vi "Configure Trigger Source.vi"(5 "Trigger Holdoff (0)":dbl min=0.0 max=1.0, 6 "Trigger Slope (0: Negative)":u16(ring) items=["Negative", "Positive", "Either"], 7 "Trigger Delay (0)":dbl min=0.0 max=10.0, 8 "error in (no error)":errorcluster, 9 "Trigger State (2: Idle)":u16(ring)=2 items=["Single", "Continuous", "Idle"], 10 "Source (0: Bus)":u16(ring) items=["Bus", "External", "Hold"], 11 "VISA resource name":refnum<visa-resource-name>) -> (0 "error out":errorcluster, 3 "VISA resource name out":refnum<visa-resource-name>)   [LabVIEW 2017, in "HH PLI Series.lvlib"]
doc: "Configures trigger event source, slope trigger delay time and trigger holdoff time.\nInitiates trigger system after configuration if <b>Trigger State</b> is set to Single or Continuous.\n\n<b>Note</b>\nSlope is only relevant for external source."
uses:
  HH PLI Series.lvlib
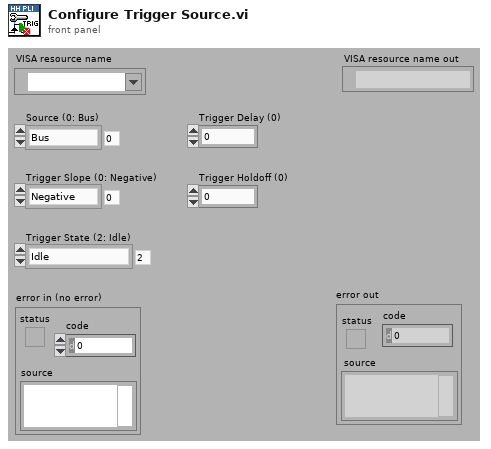
[diagram p1: front panel]
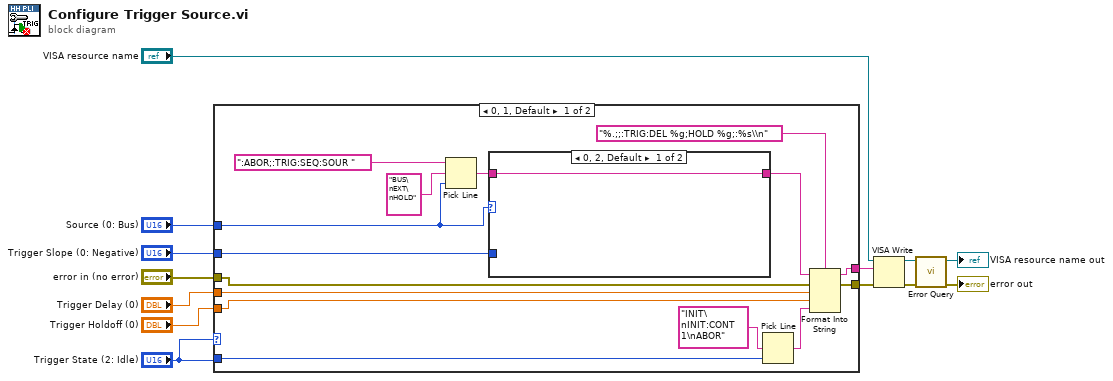
[diagram p0: block diagram]
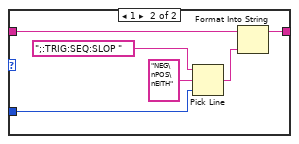
[diagram p2: hidden frame]
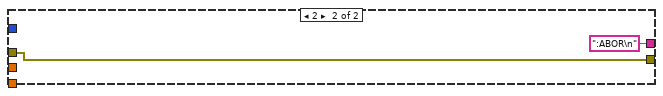
[diagram p3: hidden frame]
diagram:
  n1 = case shown="0, 1, Default" "Trigger State (2: Idle)" {
    tunnel: "Source (0: Bus)" -> [w26 _]
    tunnel: "Trigger Slope (0: Negative)" -> [w24 _]
    tunnel: "Trigger State (2: Idle)" -> [w22 _]
    tunnel: [w20 ":ABOR\n"] -> w6
    tunnel: "Trigger Holdoff (0)" -> [w16 _]
    tunnel: "Trigger Delay (0)" -> [w18 _]
    tunnel: [w15 w36] -> w2
    tunnel: "error in (no error)" -> [w14 w36]
    frame 0, 1, Default {
      n2 = Pick Line(string ("")=":ABOR;:TRIG:SEQ:SOUR " ("command"), multi-line string="BUS\nEXT\nHOLD", line index=w26) -> (output string=w25:string)
      n3 = case shown="0, 2, Default" w26 {
        tunnel: [w29 w30] -> w21
        tunnel: w25 -> [w29 w32]
        tunnel: w24 -> [_ w33]
        frame 0, 2, Default {
        }
        frame 1 {
          n4 = Pick Line(string ("")=";:TRIG:SEQ:SLOP " ("command"), multi-line string="NEG\nPOS\nEITH", line index=w33) -> (output string=w31:string)
          n5 = Format Into String(initial string=w32, w31) -> (resulting string=w30:string)  [unwired: 2 in, 1 out]
        }
      }
      n6 = Pick Line(multi-line string="INIT\nINIT:CONT 1\nABOR" ("command"), line index=w22) -> (output string=w17:string)  [unwired: 1 in]
      n7 = Format Into String(format string="%.;;:TRIG:DEL %g;HOLD %g;:%s\\n", initial string=w21, error in=w14, w18, w16, w17) -> (resulting string=w20:string, error out=w15:errorcluster)
    }
    frame 2 {
    }
  }
  n8 = VISA Write(VISA resource name="VISA resource name", write buffer=w6, error in (no error)=w2) -> (VISA resource name out=w11:refnum<visa-resource-name>, error out=w12:errorcluster)  [unwired: 1 out]
  n9 = call "Error Query.vi"("error in (no error)"=w12, "VISA resource name"=w11) -> ("error out"=→"error out":errorcluster, "VISA resource name out"=→"VISA resource name out":refnum<visa-resource-name>)  [unwired: 6 in, 2 out]
